vi "Close Connections.vi"(8 "error in (no error)":errorcluster, 11 "Interlock Chain in":refnum<class "Interlock Chain.lvclass">) -> (0 "error out":errorcluster, 3 "Interlock Chain out":refnum<class "Interlock Chain.lvclass">)   [LabVIEW 2015, in "Interlocks.lvlib" / "Interlock Chain.lvclass"]
uses:
  Interlock Chain.lvclass
  Interlock Chain.lvclass/Interlock Chain.ctl
  Interlock/Interlock.lvclass
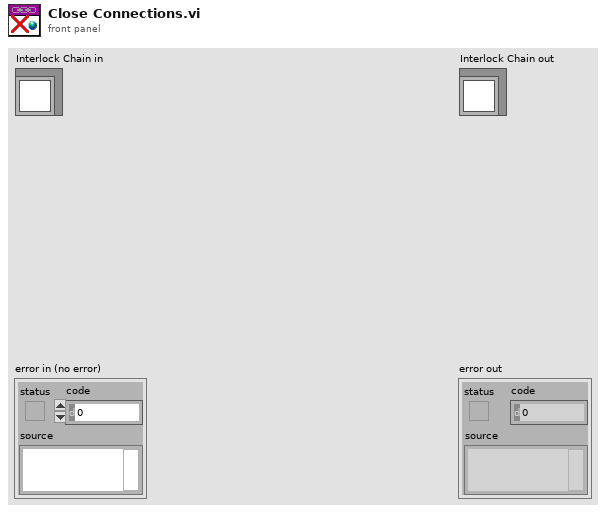
[diagram p1: front panel]
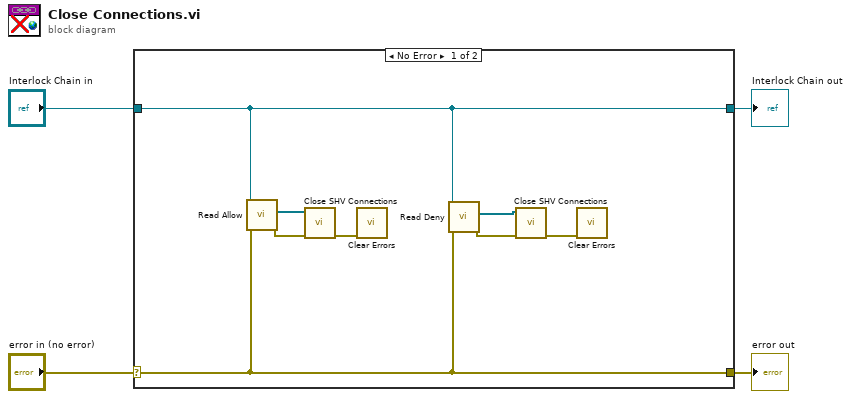
[diagram p0: block diagram]
diagram:
  n1 = case shown="No Error" "error in (no error)" {
    selector: "error in (no error)" -> [w11 w14]
    tunnel: [w11 w14] -> w3
    tunnel: [w12 w13] -> w1
    tunnel: "Interlock Chain in" -> [w12 w13]
    frame No Error {
      n2 = call "Read Allow.vi"("error in (no error)"=w11, "Interlock Chain in"=w12) -> ("error out"=w9:errorcluster, "Allow"=w10:refnum<class "Interlock.lvclass">[])  [unwired: 6 in, 2 out]
      n3 = call "Close SHV Connections.vi"("error in (no error)"=w9, "Interlocks in"=w10) -> ("error out"=w6:errorcluster)  [unwired: 8 in, 1 out]
      n4 = call <vilib>:"Clear Errors.vi"("error in (no error)"=w6) -> ()  [unwired: 5 in, 2 out]
      n5 = call "Read Deny.vi"("error in (no error)"=w11, "Interlock Chain in"=w12) -> ("error out"=w7:errorcluster, "Deny"=w8:refnum<class "Interlock.lvclass">[])  [unwired: 7 in, 1 out]
      n6 = call "Close SHV Connections.vi"("error in (no error)"=w7, "Interlocks in"=w8) -> ("error out"=w5:errorcluster)  [unwired: 8 in, 1 out]
      n7 = call <vilib>:"Clear Errors.vi"("error in (no error)"=w5) -> ()  [unwired: 5 in, 2 out]
    }
    frame Error {
    }
  }
  "error out" <- w3
  "Interlock Chain out" <- w1
